vi "InPutMAP.vi"(8 "error in (no error)":errorcluster, 10 "Notifiers.Control":T2, 11 "Mapping Buss In":T3) -> (0 "error out":errorcluster, 1 "HW CTRL Data":T1)   [LabVIEW 2014, in "SeqLoop.lvlib"]
uses:
  SeqLoop.lvlib
  TypeDefs/HW InOut MAP.ctl
  APIs/Data Queue/Control Data Cluster.ctl
  TypeDefs/HW CTRL Data.ctl
  APIs/Data Queue/WINFAS 2 Data Queue.lvlib
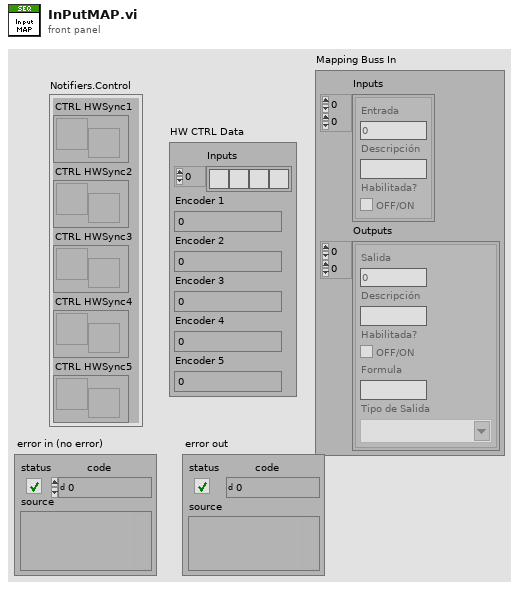
[diagram p1: front panel]
types:
  T1 = typedef "SeqLoop.lvlib/HW CTRL Data.ctl" = cluster{"Inputs":bool[], "Encoder 1":sgl, "Encoder 2":sgl, "Encoder 3":sgl, "Encoder 4":sgl, "Encoder 5":sgl}
  T2 = cluster{"CTRL HWSync1":refnum<notifier>, "CTRL HWSync2":refnum<notifier>, "CTRL HWSync3":refnum<notifier>, "CTRL HWSync4":refnum<notifier>, "CTRL HWSync5":refnum<notifier>}
  T3 = typedef "SeqLoop.lvlib/HW InOut MAP.ctl" = cluster{"Inputs":cluster{"Entrada":i32, "Descripción":string, "Habilitada?":bool}[][], "Outputs":cluster{"Salida":i32, "Descripción":string, "Habilitada?":bool, "Formula":string, "Tipo de Salida":string}[][]}
  T4 = typedef "WINFAS 2 Data Queue.lvlib/Control Data Cluster.ctl" = cluster{"Encoder":sgl, "DI":bool[], "DO":bool[]}
  T5 = cluster{"Entrada":i32, "Descripción":string, "Habilitada?":bool}[][]
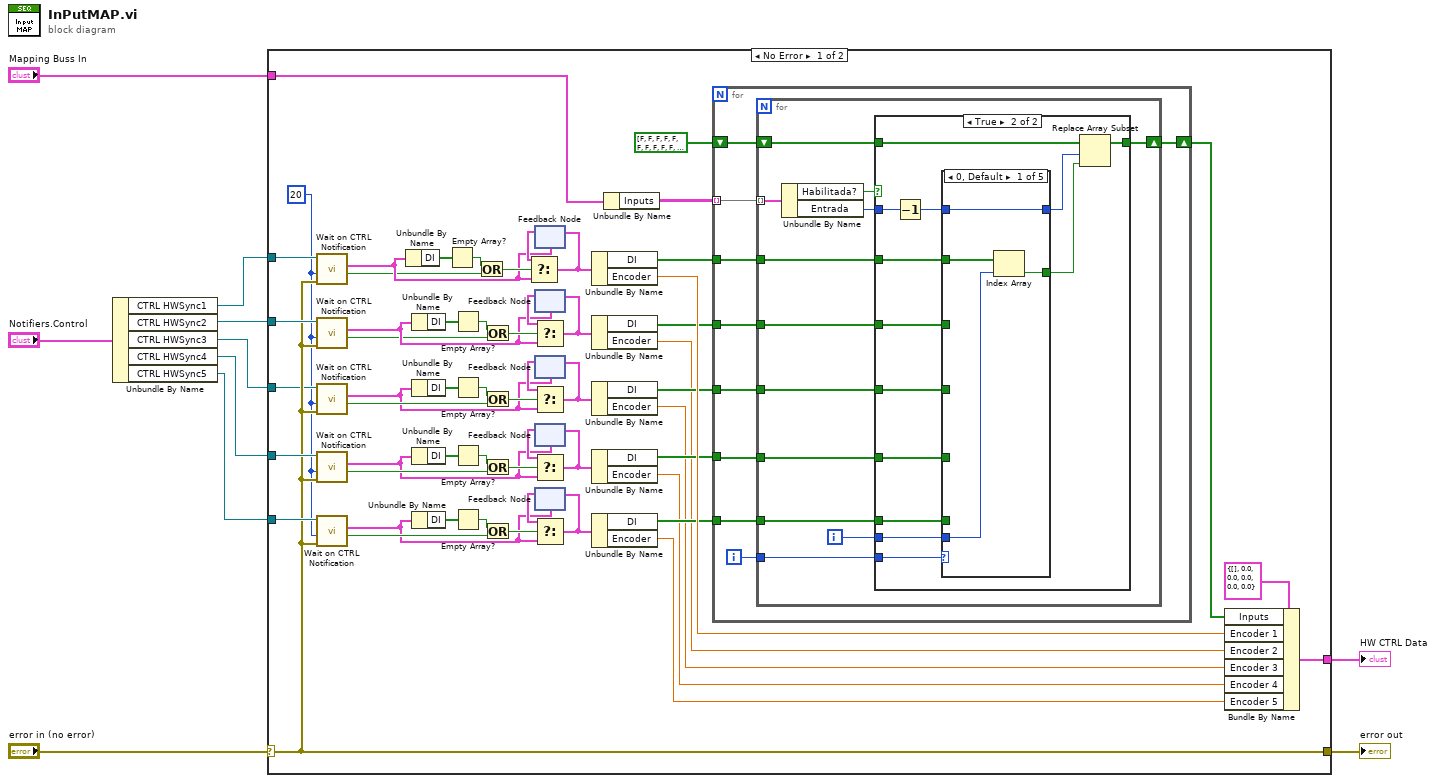
[diagram p0: block diagram]
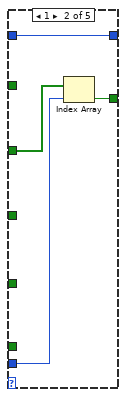
[diagram p3: hidden frame]
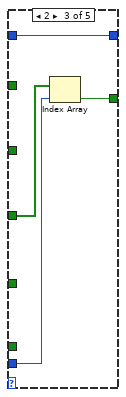
[diagram p4: hidden frame]
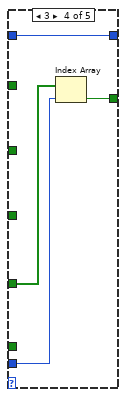
[diagram p5: hidden frame]
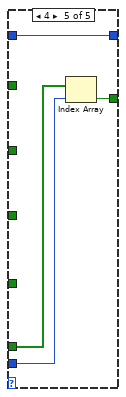
[diagram p6: hidden frame]
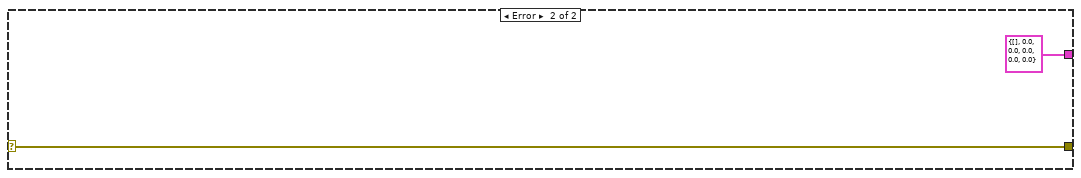
[diagram p7: hidden frame]
diagram:
  n1 = Unbundle By Name("Notifiers.Control") -> ("CTRL HWSync1"=w7:refnum<notifier>, "CTRL HWSync2"=w6:refnum<notifier>, "CTRL HWSync3"=w5:refnum<notifier>, "CTRL HWSync4"=w4:refnum<notifier>, "CTRL HWSync5"=w3:refnum<notifier>)
  n2 = case shown="No Error" "error in (no error)" {
    selector: "error in (no error)" -> [w58 w125]
    tunnel: "Mapping Buss In" -> [w66 _]
    tunnel: [w58 w125] -> w8
    tunnel: w7 -> [w65 _]
    tunnel: w6 -> [w64 _]
    tunnel: w5 -> [w12 _]
    tunnel: w4 -> [w63 _]
    tunnel: w3 -> [w62 _]
    tunnel: [w60 T1 {"Inputs"=[], "Encoder 1"=0.0, "Encoder 2"=0.0, "Encoder 3"=0.0, "Encoder 4"=0.0, "Encoder 5"=0.0} ("Logic Variable Data 2")] -> w2
    frame No Error {
      w11 = 20 ("timeout in ms (-1)")
      n3 = call "Wait on CTRL Notification.vi"("error in (no error)"=w58, "timeout in ms (-1)"=w11, "CTRL Data Notifier in"=w65) -> ("timed out?"=w49:bool, "Control Data"=w52:T4)  [unwired: 5 in, 2 out]
      n4 = call "Wait on CTRL Notification.vi"("error in (no error)"=w58, "timeout in ms (-1)"=w11, "CTRL Data Notifier in"=w64) -> ("timed out?"=w13:bool, "Control Data"=w23:T4)  [unwired: 5 in, 2 out]
      n5 = call "Wait on CTRL Notification.vi"("error in (no error)"=w58, "timeout in ms (-1)"=w11, "CTRL Data Notifier in"=w12) -> ("timed out?"=w26:bool, "Control Data"=w22:T4)  [unwired: 5 in, 2 out]
      n6 = call "Wait on CTRL Notification.vi"("error in (no error)"=w58, "timeout in ms (-1)"=w11, "CTRL Data Notifier in"=w63) -> ("timed out?"=w27:bool, "Control Data"=w21:T4)  [unwired: 5 in, 2 out]
      n7 = call "Wait on CTRL Notification.vi"("error in (no error)"=w58, "timeout in ms (-1)"=w11, "CTRL Data Notifier in"=w62) -> ("timed out?"=w28:bool, "Control Data"=w20:T4)  [unwired: 5 in, 2 out]
      n8 = Unbundle By Name(w52) -> ("DI"=w54:bool[])
      n9 = Unbundle By Name(w23) -> ("DI"=w47:bool[])
      n10 = Unbundle By Name(w22) -> ("DI"=w40:bool[])
      n11 = Unbundle By Name(w21) -> ("DI"=w37:bool[])
      n12 = Unbundle By Name(w20) -> ("DI"=w30:bool[])
      n13 = Empty Array?(array=w54) -> (empty?=w55:bool)
      n14 = Empty Array?(array=w47) -> (empty?=w46:bool)
      n15 = Empty Array?(array=w40) -> (empty?=w41:bool)
      n16 = Empty Array?(array=w37) -> (empty?=w36:bool)
      n17 = Empty Array?(array=w30) -> (empty?=w31:bool)
      n18 = Or(x=w55, y=w49) -> (x .or. y?=w53:bool)
      n19 = Or(x=w46, y=w13) -> (x .or. y?=w48:bool)
      n20 = Or(x=w41, y=w26) -> (x .or. y?=w39:bool)
      n21 = Or(x=w36, y=w27) -> (x .or. y?=w38:bool)
      n22 = Or(x=w31, y=w28) -> (x .or. y?=w29:bool)
      n23 = feedback #1(w52) -> (w57:T4)
      n24 = Select(t=w57, s=w53, f=w52) -> (s? t:f=w56:T4)
      n25 = feedback-in #1(w56) -> ()
      n26 = feedback #2(w23) -> (w44:T4)
      n27 = Select(t=w44, s=w48, f=w23) -> (s? t:f=w45:T4)
      n28 = feedback-in #2(w45) -> ()
      n29 = feedback #3(w22) -> (w43:T4)
      n30 = Select(t=w43, s=w39, f=w22) -> (s? t:f=w42:T4)
      n31 = feedback-in #3(w42) -> ()
      n32 = feedback #4(w21) -> (w34:T4)
      n33 = Select(t=w34, s=w38, f=w21) -> (s? t:f=w35:T4)
      n34 = feedback-in #4(w35) -> ()
      n35 = feedback #5(w20) -> (w33:T4)
      n36 = Select(t=w33, s=w29, f=w20) -> (s? t:f=w32:T4)
      n37 = feedback-in #5(w32) -> ()
      n38 = Unbundle By Name(w56) -> ("DI"=w51:bool[], "Encoder"=w50:sgl)
      n39 = Unbundle By Name(w45) -> ("DI"=w18:bool[], "Encoder"=w17:sgl)
      n40 = Unbundle By Name(w42) -> ("DI"=w25:bool[], "Encoder"=w16:sgl)
      n41 = Unbundle By Name(w35) -> ("DI"=w24:bool[], "Encoder"=w15:sgl)
      n42 = Unbundle By Name(w32) -> ("DI"=w19:bool[], "Encoder"=w14:sgl)
      n43 = Unbundle By Name(w66) -> ("Inputs"=w68:T5)
      n44 = for {
        tunnel: w68 -> [w76] mode=indexing
        tunnel: w51 -> [w77]
        tunnel: w18 -> [w74]
        tunnel: w25 -> [w73]
        tunnel: w24 -> [w72]
        tunnel: w19 -> [w71]
        shift-right: [w69] -> w59
        shift-left: bool[] [FALSE, FALSE, FALSE, FALSE, FALSE, FALSE, FALSE, FALSE, FALSE, FALSE, FALSE, FALSE, FALSE, FALSE, FALSE, FALSE, FALSE, FALSE, FALSE, FALSE, FALSE, FALSE, FALSE, FALSE, FALSE, FALSE, FALSE, FALSE, FALSE, FALSE, FALSE, FALSE, FALSE] ("DI") -> [w70]
        i -> [w75]
        n45 = for {
          tunnel: w76 -> [w83] mode=indexing
          tunnel: w77 -> [w88]
          tunnel: w75 -> [w89]
          tunnel: w74 -> [w87]
          tunnel: w73 -> [w86]
          tunnel: w72 -> [w85]
          tunnel: w71 -> [w84]
          shift-right: [w80] -> w69
          shift-left: w70 -> [w81]
          i -> [w82]
          n46 = Unbundle By Name(w83) -> ("Habilitada?"=w78:bool, "Entrada"=w79:i32)
          n47 = case shown="True" w78 {
            tunnel: w89 -> [_ w103]
            tunnel: w88 -> [_ w102]
            tunnel: w87 -> [_ w101]
            tunnel: w86 -> [_ w100]
            tunnel: w85 -> [_ w99]
            tunnel: w84 -> [_ w98]
            tunnel: w82 -> [_ w91]
            tunnel: w81 -> [w90 w96]
            tunnel: [w90 w95] -> w80
            tunnel: w79 -> [_ w92]
            frame False {
            }
            frame True {
              n48 = Decrement(x=w92) -> (x-1=w93:i32)
              n49 = case shown="0, Default" w103 {
                tunnel: w102 -> [w106 _ _ _ _]
                tunnel: w101 -> [_ w110 _ _ _]
                tunnel: w100 -> [_ _ w114 _ _]
                tunnel: w99 -> [_ _ _ w118 _]
                tunnel: w98 -> [_ _ _ _ w122]
                tunnel: w93 -> [w107 w111 w115 w119 w123]
                tunnel: w91 -> [w105 w109 w113 w116 w121]
                tunnel: [w107 w111 w115 w119 w123] -> w97
                tunnel: [w104 w108 w112 w117 w120] -> w94
                frame 0, Default {
                  n50 = Index Array(array=w106, index=w105) -> (element=w104:bool)
                }
                frame 1 {
                  n51 = Index Array(array=w110, index=w109) -> (element=w108:bool)
                }
                frame 2 {
                  n52 = Index Array(array=w114, index=w113) -> (element=w112:bool)
                }
                frame 3 {
                  n53 = Index Array(array=w118, index=w116) -> (element=w117:bool)
                }
                frame 4 {
                  n54 = Index Array(array=w122, index=w121) -> (element=w120:bool)
                }
              }
              n55 = Replace Array Subset(array=w96, new element=w94, index=w97) -> (w95:bool[])
            }
          }
        }
      }
      n56 = Bundle By Name(cluster=T1 {"Inputs"=[], "Encoder 1"=0.0, "Encoder 2"=0.0, "Encoder 3"=0.0, "Encoder 4"=0.0, "Encoder 5"=0.0} ("Logic Variable Data 2"), "Inputs"=w59, "Encoder 1"=w50, "Encoder 2"=w17, "Encoder 3"=w16, "Encoder 4"=w15, "Encoder 5"=w14) -> (w60:T1)
    }
    frame Error {
    }
  }
  "error out" <- w8
  "HW CTRL Data" <- w2
